vi "Create Map.vi"(8 "error in (no error)":errorcluster, 11 "Edit.Subpanel in":refnum<class "Subpanel.Edit.lvclass">) -> (0 "error out":errorcluster, 3 "Edit.Subpanel out":refnum<class "Subpanel.Edit.lvclass">)   [LabVIEW 2019, in "Subpanel.Edit.lvclass"]
uses:
  Subpanel.Edit.lvclass
  Edit/Edit.Path/Edit.Path.lvclass
  C:/Program Files (x86)/National Instruments/LabVIEW 2019/vi.lib/JKI/JKI SMO/SMO/SMO.lvclass
  C:/Users/Albro/Documents/GitHub/AFM-Lithography/lvsrc/Classes/Subpanel/Edit/Edit/Edit.lvclass
  Edit/Edit/Edit.lvclass
  Edit/Edit.Rect/Edit.Rect.lvclass
  Edit/Edit.Funnel/Edit.Funnel.lvclass
  Edit/Edit.Dot/Edit.Dot.lvclass
  Subpanel.Edit.lvclass/Subpanel.Edit.ctl
  <vilib>/JKI/JKI SMO/SMO/SMO.lvclass
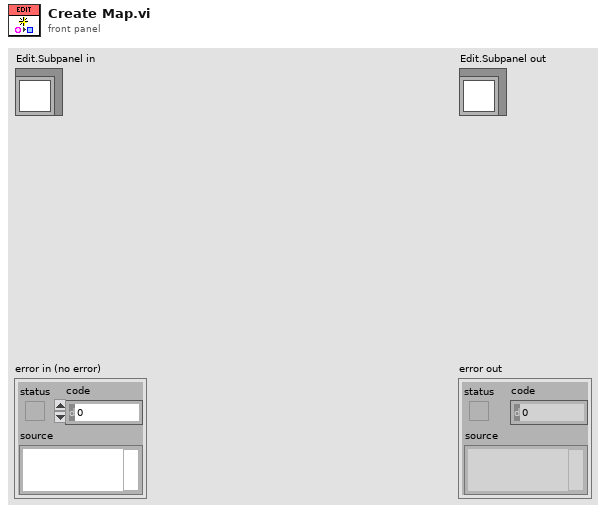
[diagram p1: front panel]
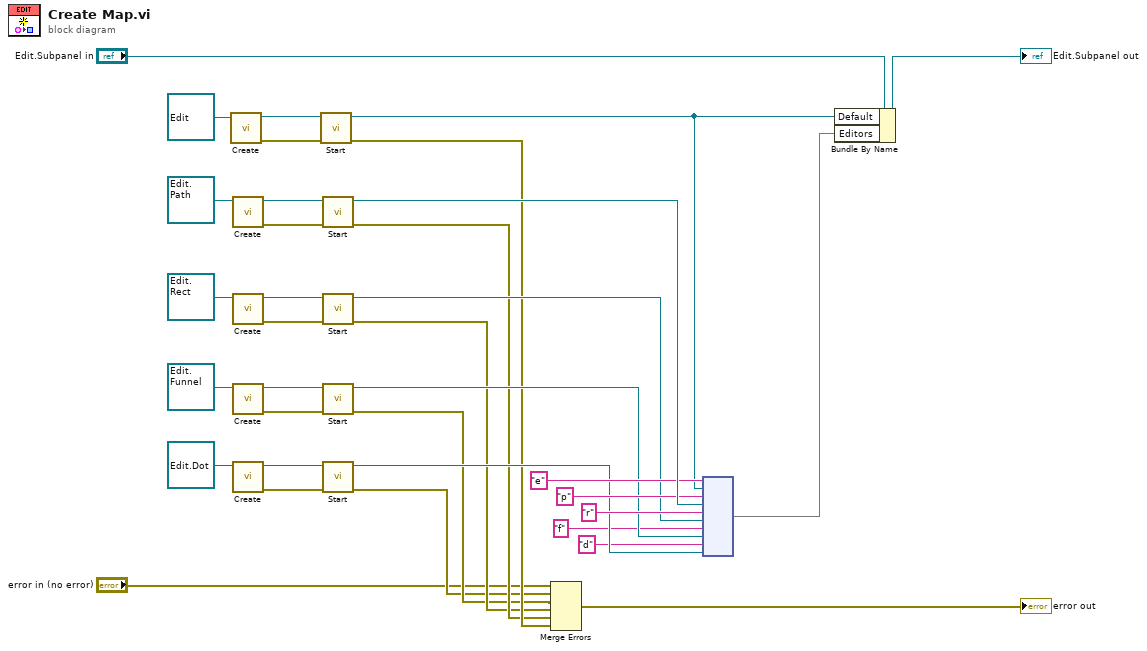
[diagram p0: block diagram]
diagram:
  n1 = call <vilib>:"Create.vi"("SMO"=refnum<class "Edit.lvclass"> refnum ("Edit.lvclass")) -> ("error out"=w27:errorcluster, "SMO out"=w34:refnum<class "Edit.lvclass">)  [unwired: 8 in, 1 out]
  n2 = call <vilib>:"Create.vi"("SMO"=refnum<class "Edit.Path.lvclass"> refnum ("Edit.Path.lvclass")) -> ("error out"=w28:errorcluster, "SMO out"=w33:refnum<class "Edit.Path.lvclass">)  [unwired: 8 in, 1 out]
  n3 = call <vilib>:"Create.vi"("SMO"=refnum<class "Edit.Rect.lvclass"> refnum ("Edit.Rect.lvclass")) -> ("error out"=w26:errorcluster, "SMO out"=w25:refnum<class "Edit.Rect.lvclass">)  [unwired: 8 in, 1 out]
  n4 = call <vilib>:"Create.vi"("SMO"=refnum<class "Edit.Funnel.lvclass"> refnum ("Edit.Funnel.lvclass")) -> ("error out"=w20:errorcluster, "SMO out"=w21:refnum<class "Edit.Funnel.lvclass">)  [unwired: 8 in, 1 out]
  n5 = call <vilib>:"Create.vi"("SMO"=refnum<class "Edit.Dot.lvclass"> refnum ("Edit.Dot.lvclass")) -> ("error out"=w19:errorcluster, "SMO out"=w18:refnum<class "Edit.Dot.lvclass">)  [unwired: 8 in, 1 out]
  n6 = call <vilib>:"Start.vi"("error in (no error)"=w27, "SMO"=w34) -> ("error out"=w11:errorcluster, "SMO out"=w2:refnum<class "Edit.lvclass">)  [unwired: 8 in]
  n7 = call <vilib>:"Start.vi"("error in (no error)"=w28, "SMO"=w33) -> ("error out"=w10:errorcluster, "SMO out"=w31:refnum<class "Edit.Path.lvclass">)  [unwired: 8 in]
  n8 = call <vilib>:"Start.vi"("error in (no error)"=w26, "SMO"=w25) -> ("error out"=w9:errorcluster, "SMO out"=w22:refnum<class "Edit.Rect.lvclass">)  [unwired: 8 in]
  n9 = call <vilib>:"Start.vi"("error in (no error)"=w20, "SMO"=w21) -> ("error out"=w8:errorcluster, "SMO out"=w17:refnum<class "Edit.Funnel.lvclass">)  [unwired: 8 in]
  n10 = call <vilib>:"Start.vi"("error in (no error)"=w19, "SMO"=w18) -> ("error out"=w7:errorcluster, "SMO out"=w16:refnum<class "Edit.Dot.lvclass">)  [unwired: 8 in]
  n11 = Merge Errors("error in (no error)", w7, w8, w9, w10, w11) -> (→"error out":errorcluster)
  n12 = node("e" ("key"), w2, "p" ("key"), w31, "r" ("key"), w22, "f" ("key"), w17, "d" ("key"), w16) -> (w1:map{string, refnum<class "Edit.lvclass">})
  n13 = Bundle By Name(cluster="Edit.Subpanel in", "Default"=w2, "Editors"=w1) -> (→"Edit.Subpanel out":refnum<class "Subpanel.Edit.lvclass">)
